vi "Data Logger DS18x20 to LCD_SD Card.vi"() -> ()   [LabVIEW 2014]
doc: "This example shows how to created a completed temperature data logger application. first it's will read temp data from DS12b20 sensor, then display the value at LCD 16x2 display and finally logging current date/time from RTC with temp data to SD Card."
uses:
  <vilib>/Aledyne-TSXperts/Arduino Compatible Compiler for LabVIEW/Code Generator/Arduino APIs/I2C LCD/LiquidCrystal_I2C write String.vi
  <vilib>/Aledyne-TSXperts/Arduino Compatible Compiler for LabVIEW/Arduino Compatible Compiler for LabVIEW.lvlib
  PWS_ESP8266/PWS_ESP8266.lvlib
  QwaveSys_Interface/QwaveSys_Interface.lvlib
panel:
  in  "DS18x20 Pin":u8(ring)=15 items=["SPI#1/SS,(5)"=5, "SPI#2/MOSI,(13)"=13, "SPI#3/MISO,(12)"=12, "SPI#4/SCLK,(14)"=14, "UART#1/CS,(15)"=15, "UART#2/TXD,(1)"=1, "UART#3/RXD,(3)"=3, "UART#4/LED,(16)"=16, "FPROM_Btn,(0)"=0, "SDCard_CS,(4)"=4, "I2C-SDA/TXD1,(2)"=2, "ADC0,(17)"=17]
  # "Overview: Demonstrates how to create temperature data logger application using  DS18b20 sensor connected to digital pin, then display value at 16x2 LCD screen after that continue logging time/date data & temperature data to internal SD card.\nRequirements: LabVIEW Full Development System,Arduino Compatible Compiler for LabVIEW,Programmable Wireless Stamp (PWS) Library.\nInstructions:\n1. Wire a temperature sensor DS18x20 (This example using DS18b20) as specified below where the data pin is wired to the specified Digital Pin (GPIO15) below.\n2. Wire the LCD's power pins to VCC and GND and the I2C pins to the Pmod I2C interface.  Note that on an PWS board, the I2C pins are on GPIO2 (SDA) and GPIO14 (SCL) \n3. Insert uSD card into micro SD card slot.\n4. If this example has been loaded from the Arduino Compatible Compiler for LabVIEW, simply select Compile and Download.  Otherwise, open Tools>Arduino Compatible Compiler for LabVIEW in LabVIEW, then select File>Load VI, and select this VI and then Compile and Download.\n5. Observe the date/time and temperature data being written to the LCD.\n6. Open \"Serial Monitor\" by select \"Tools>Serial Monitor\" and select baud rate to 9600.\n7. Observe the logged data being print out on serial port monitor. \n8. Removed uSD card and open it via PC, Observed \"DSLog.csv\" log file inside uSD card, This .csv file can be open using Notepad or Microsoft Excel for data analysis purpose."
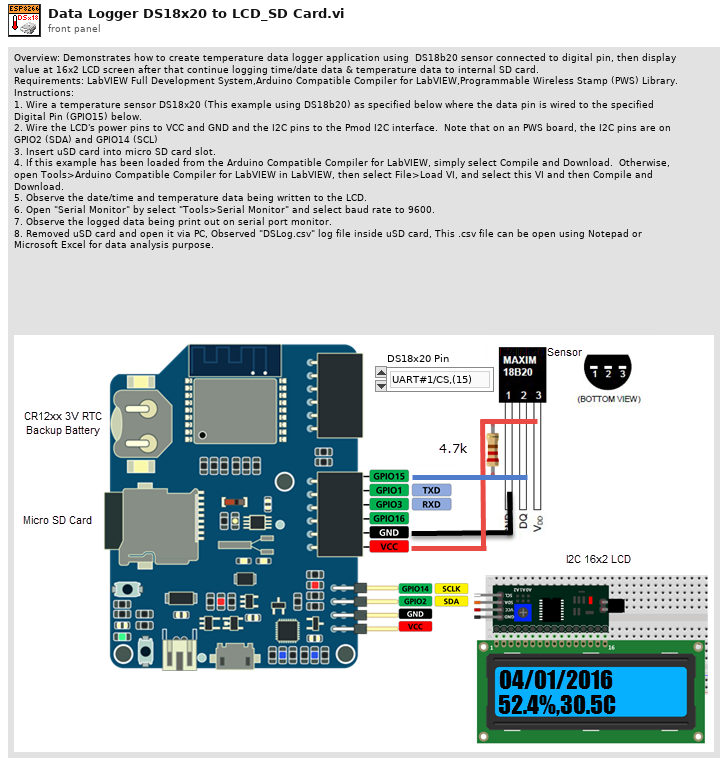
[diagram p1: front panel]
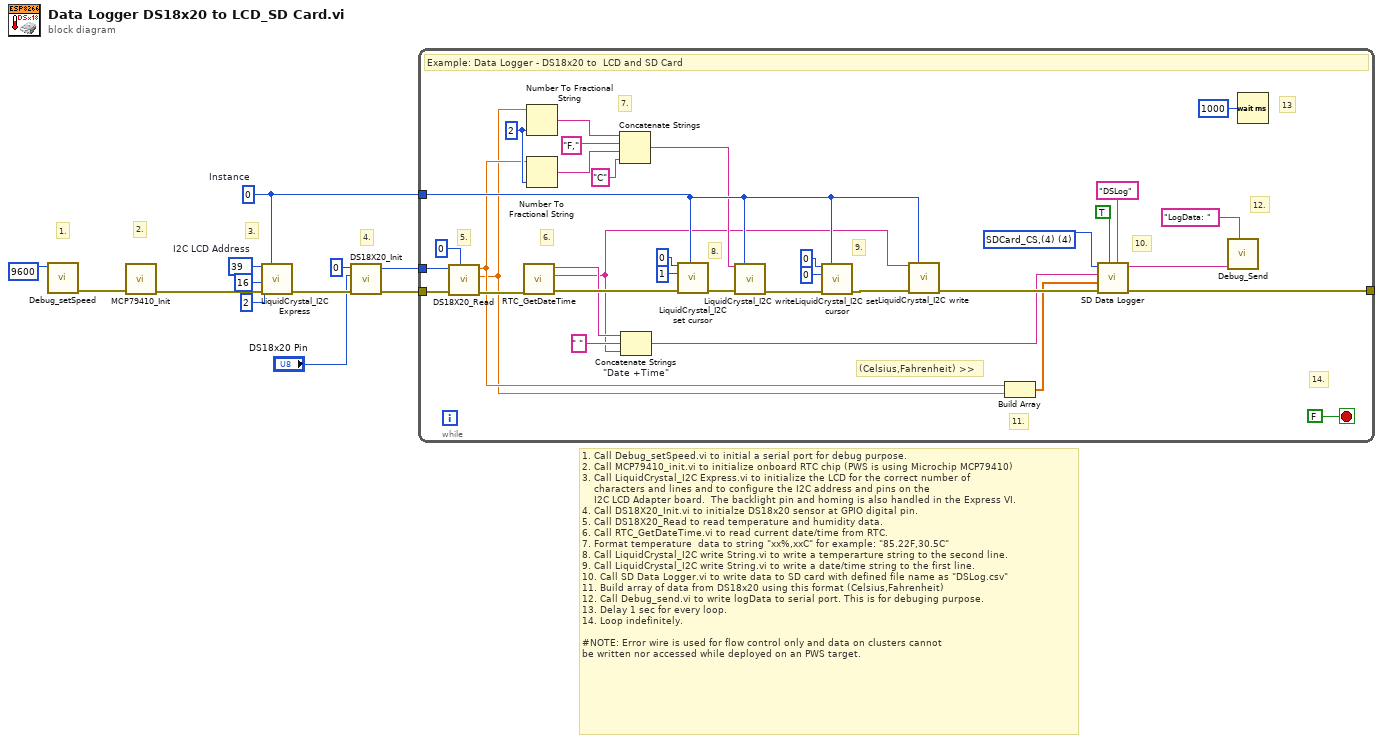
[diagram p0: block diagram]
diagram:
  w12 = u8 39  # I2C LCD Address
  w9 = u8 0  # Instance
  # "4."
  # "3."
  # "2."
  # "1."
  # "1. Call Debug_setSpeed.vi to initial a serial port for debug purpose.\n2. Call MCP79410_init.vi to initialize onboard RTC chip (PWS is using Microchip MCP79410)\n3. Call LiquidCrystal_I2C Express.vi to initialize the LCD for the correct number of\n    characters and lines and to configure the I2C address and pins on the\n    I2C LCD Adapter board.  The backlight pin and homing is also handled in the Express VI.\n4. Call DS18X20_Init.vi to initialze DS18x20 sensor at GPIO digital pin. \n5. Call DS18X20_Read to read temperature and humidity data.\n6. Call RTC_GetDateTime.vi to read current date/time from RTC.\n7. Format temperature  data to string \"xx%,xxC\" for example: \"85.22F,30.5C\"\n8. Call LiquidCrystal_I2C write String.vi to write a temperarture string to the second line.\n9. Call LiquidCrystal_I2C write String.vi to write a date/time string to the first line.\n10. Call SD Data Logger.vi to write data to SD card with defined file name as \"DSLog.csv\"\n11. Build array of data from DS18x20 using this format (Celsius,Fahrenheit) \n12. Call Debug_send.vi to write logData to serial port. This is for debuging purpose.\n13. Delay 1 sec for every loop.\n14. Loop indefinitely.\n\n#NOTE: Error wire is used for flow control only and data on clusters cannot\nbe written nor accessed while deployed on an PWS target."
  n1 = call "Debug_setSpeed.vi"("Speed"=u32 9600) -> ("error out"=w7:errorcluster)  [unwired: 10 in]
  n2 = call "MCP79410_Init.vi"("error in (no error)"=w7) -> ("error out"=w6:errorcluster)  [unwired: 10 in]
  n3 = call <vilib>:"LiquidCrystal_I2C Express.vi"("Addr"=w12, "Instance"=w9, "Chars"=u16 16, "Lines"=u16 2, "error in (no error)"=w6) -> ("error out"=w5:errorcluster)  [unwired: 10 in]
  n4 = call "DS18X20_Init.vi"("error in"=w5, "PIN"="DS18x20 Pin", "Interface (0-4)"=u8 0) -> ("error out"=w4:errorcluster, "Instance"=w3:u8)  [unwired: 7 in]
  n5 = while {
    tunnel: w9 -> [w37]
    tunnel: [w31] -> _
    tunnel: w4 -> [w19]
    tunnel: w3 -> [w18]
    stop <- FALSE stop-if-true
    w23 = i16 2 ("precision (6)")
    w30 = u8 4 items=["SPI#1/SS,(5)"=5, "SPI#2/MOSI,(13)"=13, "SPI#3/MISO,(12)"=12, "SPI#4/SCLK,(14)"=14, "UART#1/CS,(15)"=15, "UART#2/TXD,(1)"=1, "UART#3/RXD,(3)"=3, "UART#4/LED,(16)"=16, "FPROM_Btn,(0)"=0, "SDCard_CS,(4)"=4, "I2C-SDA/TXD1,(2)"=2, "ADC0,(17)"=17] ("SD Card CS")
    # "14."
    # "13"
    # "12."
    # "11."
    # "10."
    # "9."
    # "8."
    # "7."
    # "6."
    # "5."
    # "(Celsius,Fahrenheit) >>"
    # "Example: Data Logger - DS18x20 to  LCD and SD Card"
    n6 = call "DS18X20_Read.vi"("Index"=i8 0, "error in (no error)"=w19, "Instance"=w18) -> ("error out"=w17:errorcluster, "F"=w15:dbl, "C"=w16:dbl)  [unwired: 6 in]
    n7 = call "RTC_GetDateTime.vi"("error in (no error)"=w17) -> ("error out"=w40:errorcluster, "time string"=w24:string, "date string"=w29:string)  [unwired: 8 in]
    n8 = Number To Fractional String(number=w15, precision (6)=w23) -> (F-format string=w26:string)  [unwired: 2 in]
    n9 = Number To Fractional String(number=w16, precision (6)=w23) -> (F-format string=w21:string)  [unwired: 2 in]
    n10 = Concatenate Strings(w26, "F," ("string"), w21, "C" ("string")) -> (w25:string)
    n11 = Concatenate Strings "\"Date +Time\""(w29, " " ("string"), w24) -> (w27:string)
    n12 = call <vilib>:"LiquidCrystal_I2C set cursor.vi"("character"=u16 0, "Instance"=w37, "line"=u16 1, "error in (no error)"=w40) -> ("error out"=w39:errorcluster)  [unwired: 11 in]
    n13 = call-poly <vilib>:"LiquidCrystal_I2C write.vi"("Data"=w25, "Instance"=w37, "error in (no error)"=w39) -> ("error out"=w38:errorcluster)  [unwired: 12 in]
    n14 = call <vilib>:"LiquidCrystal_I2C set cursor.vi"("character"=u16 0, "Instance"=w37, "line"=u16 0, "error in (no error)"=w38) -> ("error out"=w45:errorcluster)  [unwired: 11 in]
    n15 = call-poly <vilib>:"LiquidCrystal_I2C write.vi"("Data"=w24, "Instance"=w37, "error in (no error)"=w45) -> ("error out"=w32:errorcluster)  [unwired: 12 in]
    n16 = Build Array(w16, w15) -> (w14:dbl[])
    n17 = call <vilib>:"SD Data Logger.vi"("File Name"="DSLog", "Append Timestamp"=TRUE, "error in (no error)"=w32, "Data"=w14, "Timestamp"=w27, "CS Pin"=w30) -> ("error out"=w31:errorcluster, "CSV Data"=w34:string)  [unwired: 4 in]
    n18 = call "Debug_Send.vi"("Name"="LogData: ", "DATA"=w34) -> ()  [unwired: 10 in]
    n19 = Wait (ms)(milliseconds to wait=u32 1000) -> ()  [unwired: 1 out]
  }
